vi "Initialize Queues and Buffers.vi"(4 "XNET Cluster":refnum<k21>, 5 "initial values":dbl[](array[numeric]), 6 "XNET Database":refnum<k21>, 7 "scaling information":T6, 8 "error in":errorcluster, 10 "stop notifier":refnum<notifier>, 11 "J1939 init data":T1={"CAN Port"="", "CAN Termination"=0, "timing"={"tb to j1939 queue timeout"=100, "j1939 to tb queue timeout"=100, "dtc loop period (ms)"=100, "CAN in loop period (ms)"=100, "process incoming queue timeout (ms)"=100, "Outgoing Write Decimation"=0, "process outgoing loop rate (ms)"=100, "periodic outgoing queue timeout (ms)"=10, "CAN out queue timeout (ms)"=100}, "database"={"BaudRate"=0, "CAN.IoMode"=0, "J1939 Network Address"=0, "Name"=0, "frames"=[]}} {"CAN Termination" items=["Off", "On"]}) -> (0 "error out":errorcluster, 3 "j1939 internals":T8={"J1939 XNET Settings"={"XNET Database"="", "XNET Cluster"="", "CAN port"="", "Baud rate [Bd]"=0, "J1939 Network Address"=0, "Name"=0, "Termination"=0}, "j1939 queues"={"Processed Outgoing"=refnum, "Process Outgoing"=refnum, "stop notifier"=refnum, "error queue"=refnum, "active dtc"=refnum, "processed inc"=refnum}, "fgv references"={"BAM Buffer"=refnum, "CM Buffer"=refnum, "CM Gen"=refnum, "BAM Gen"=refnum, "Address Claims"=refnum, "RQST"=refnum, "scaling lut"=refnum, "data lut"=refnum, "cyclic scheduler"=refnum}, "frame in"="", "frame out"="", "timing"={"tb to j1939 queue timeout"=100, "j1939 to tb queue timeout"=100, "dtc loop period (ms)"=100, "CAN in loop period (ms)"=100, "process incoming queue timeout (ms)"=100, "Outgoing Write Decimation"=0, "process outgoing loop rate (ms)"=0, "periodic outgoing queue timeout (ms)"=10, "CAN out queue timeout (ms)"=100}})   [LabVIEW 2013, in "J1939.lvlib"]
uses:
  J1939.lvlib
  API Types/Internal Data.ctl
  API Types/XNET Settings.ctl
  Users/Benjamin/Desktop/Tag bus J1939/J1939/RT Driver/J1939 Multi Packet Frame/_SubVIs/J1939 Setup Information Cluster.ctl
  API Types/CAN Outgoing Message Cluster.ctl
  Users/Benjamin/Desktop/Tag bus J1939/J1939/RT Driver/J1939 Multi Packet Frame/_SubVIs/J1939 Convert DTCs Cluster.ctl
  <vilib>/xnet/xnet.llb/XNET Frame CAN.ctl
  <vilib>/xnet/xnet.llb/XNET Frame Type CAN.ctl
  Users/Benjamin/Desktop/Tag bus J1939/J1939/RT Driver/J1939 Multi Packet Frame/_SubVIs/J1939 TP List References.ctl
  Users/Benjamin/Desktop/Tag bus J1939/J1939/RT Driver/J1939 Multi Packet Frame/_SubVIs/J1939 BAM Buffer Connections List_Ref.ctl
  Users/Benjamin/Desktop/Tag bus J1939/J1939/RT Driver/J1939 Multi Packet Frame/_SubVIs/J1939 Connection Mode Generation Connection Ref.ctl
  Users/Benjamin/Desktop/Tag bus J1939/J1939/RT Driver/J1939 Multi Packet Frame/_SubVIs/J1939 BAM Generation Connections List_Ref.ctl
  LUTs/J1939 Address Table Reference.ctl
  Users/Benjamin/Desktop/Tag bus J1939/J1939/RT Driver/J1939 Multi Packet Frame/_SubVIs/J1939 RQST Lookup Table Reference.ctl
  LUTs/J1939 Conversion Lookup Table Reference.ctl
  LUTs/J1939 Data Lookup Table Reference.ctl
  LUTs/Cyclic Frame Scheduler Lut Reference.ctl
  Configuration/TypeDefs/timing configuration.ctl
  API Types/Scaling Initialization.ctl
  Users/Benjamin/Desktop/Tag bus J1939/J1939/RT Driver/SubVIs/CD Conversion Lookup Table Parameters Cluster.ctl
  Configuration/TypeDefs/initialization data.ctl
  Configuration/TypeDefs/J1939 db.ctl
  Configuration/TypeDefs/J1939 db frame.ctl
  Configuration/TypeDefs/J1939 db signal.ctl
  <vilib>/xnet/xnet.llb/XNET Create Session (Frame Input Stream).vi
  <vilib>/xnet/xnet.llb/XNET Create Session (Frame Output Stream).vi
  <resource>/objmgr/xnet.rc
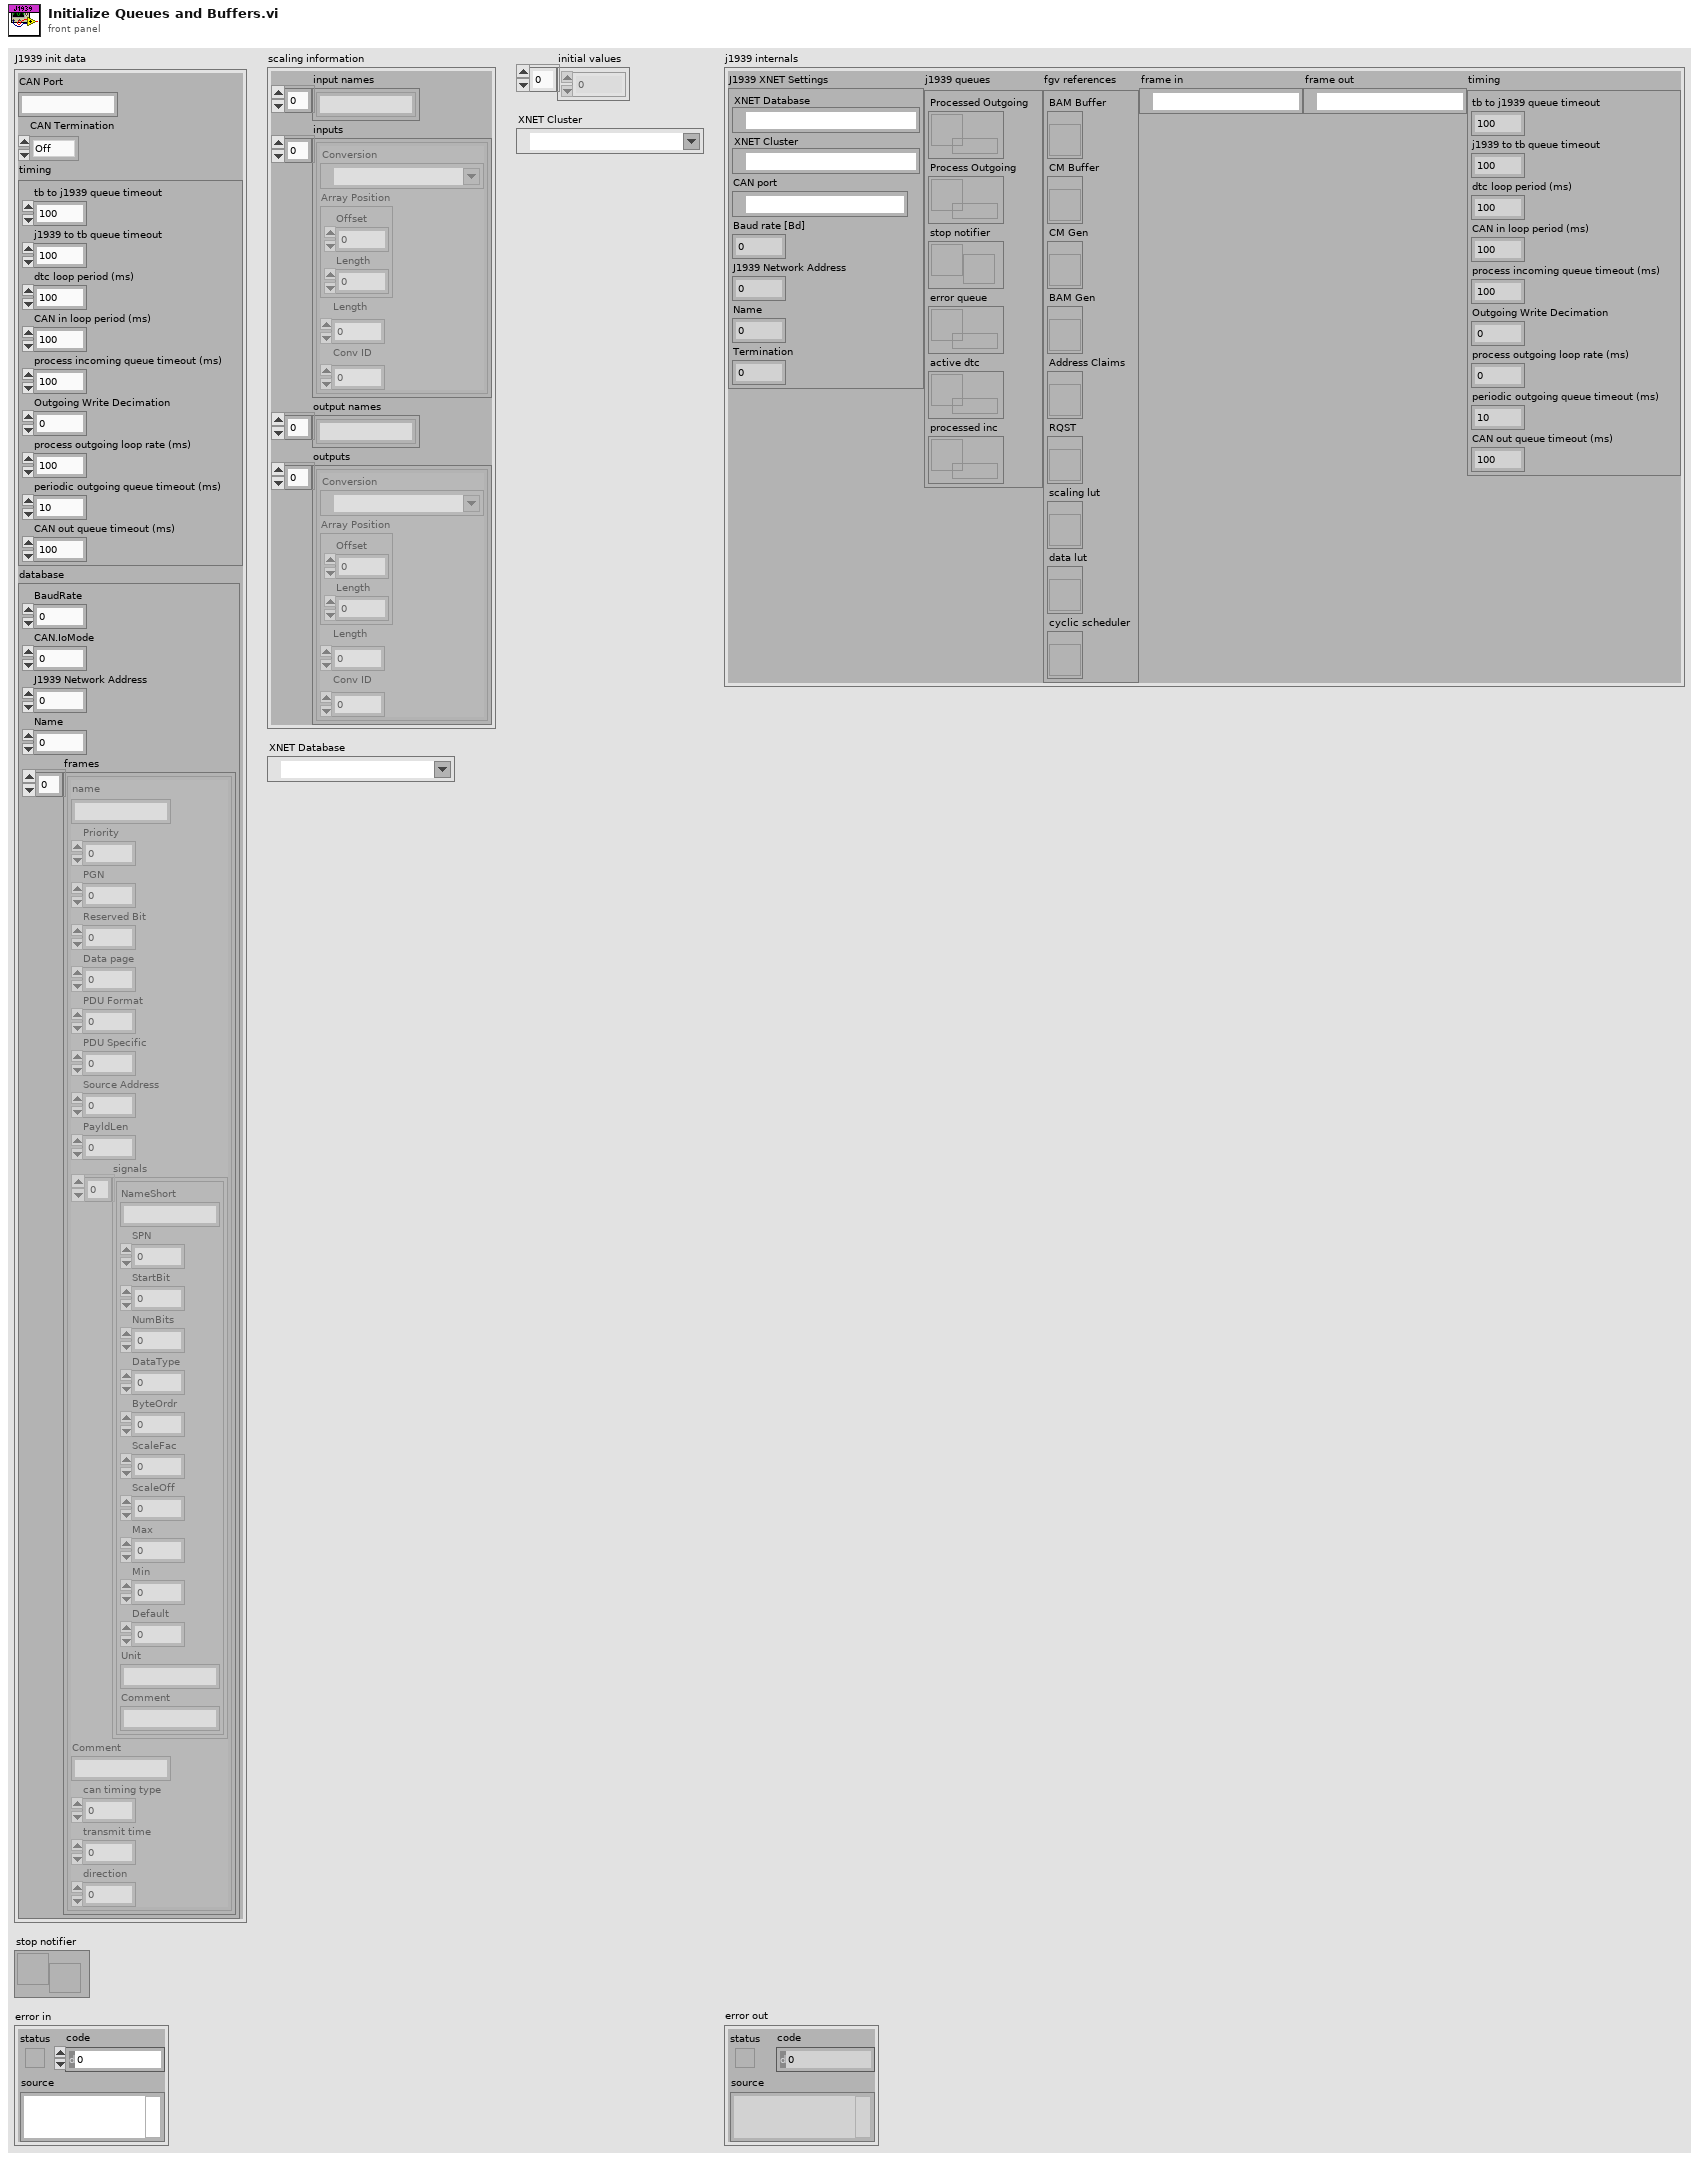
[diagram p1: front panel]
types:
  T1 = typedef "J1939.lvlib/initialization data.ctl" = cluster{"CAN Port":string, "CAN Termination":u32, "timing":T2, "database":T3}
  T2 = typedef "J1939.lvlib/timing configuration.ctl" = cluster{"tb to j1939 queue timeout":i32, "j1939 to tb queue timeout":i32, "dtc loop period (ms)":i32, "CAN in loop period (ms)":i32, "process incoming queue timeout (ms)":i32, "Outgoing Write Decimation":u32, "process outgoing loop rate (ms)":i32, "periodic outgoing queue timeout (ms)":i32, "CAN out queue timeout (ms)":i32}
  T3 = typedef "J1939.lvlib/J1939 db.ctl" = cluster{"BaudRate":u32, "CAN.IoMode":u32, "J1939 Network Address":u8, "Name":u64, "frames":T4[]}
  T4 = typedef "J1939.lvlib/J1939 db frame.ctl" = cluster{"name":string, "Priority":u8, "PGN":u32, "Reserved Bit":u8, "Data page":u8, "PDU Format":u8, "PDU Specific":u8, "Source Address":u8, "PayldLen":u32, "signals":T5[], "Comment":string, "can timing type":u32, "transmit time":dbl, "direction":u16}
  T5 = typedef "J1939.lvlib/J1939 db signal.ctl" = cluster{"NameShort":string, "SPN":i32, "StartBit":u32, "NumBits":u32, "DataType":u32, "ByteOrdr":u32, "ScaleFac":dbl, "ScaleOff":dbl, "Max":dbl, "Min":dbl, "Default":dbl, "Unit":string, "Comment":string}
  T6 = typedef "J1939.lvlib/scaling initialization.ctl" = cluster{"input names":string[], "inputs":T7[], "output names":string[], "outputs":T7[]}
  T7 = typedef "J1939.lvlib/CD Conversion Lookup Table Parameters Cluster.ctl" = cluster{"Conversion":refnum<k21>, "Array Position":cluster{"Offset":u32, "Length":u32}, "Length":u32, "Conv ID":u32}
  T8 = typedef "J1939.lvlib/Internal Data.ctl" = cluster{"J1939 XNET Settings":T9, "j1939 queues":T10, "fgv references":T11, "frame in":refnum<k21>, "frame out":refnum<k21>, "timing":T2}
  T9 = typedef "J1939.lvlib/XNET settings.ctl" = cluster{"XNET Database":refnum<k21>, "XNET Cluster":refnum<k21>, "CAN port":refnum<k21>, "Baud rate [Bd]":u32, "J1939 Network Address":u8, "Name":u64, "Termination":u32}
  T10 = typedef "J1939.lvlib/J1939 Setup Information Cluster.ctl" = cluster{"Processed Outgoing":refnum<queue>, "Process Outgoing":refnum<queue>, "stop notifier":refnum<notifier>, "error queue":refnum<queue>, "active dtc":refnum<queue>, "processed inc":refnum<queue>}
  T11 = typedef "J1939.lvlib/J1939 TP List References.ctl" = cluster{"BAM Buffer":T12, "CM Buffer":T12, "CM Gen":T13, "BAM Gen":T14, "Address Claims":T15, "RQST":T16, "scaling lut":T17, "data lut":T18, "cyclic scheduler":T19}
  T12 = typedef "J1939.lvlib/J1939 BAM Buffer Connections List_Ref.ctl" = refnum<vi>
  T13 = typedef "J1939.lvlib/J1939 Connection Mode Generation Connection Ref.ctl" = refnum<vi>
  T14 = typedef "J1939.lvlib/J1939 BAM Generation Connections List_Ref.ctl" = refnum<vi>
  T15 = typedef "J1939.lvlib/J1939 Address Table Reference.ctl" = refnum<vi>
  T16 = typedef "J1939.lvlib/J1939 RQST Lookup Table Reference.ctl" = refnum<vi>
  T17 = typedef "J1939.lvlib/J1939 Conversion Lookup Table Reference.ctl" = refnum<vi>
  T18 = typedef "J1939.lvlib/J1939 Data Lookup Table Reference.ctl" = refnum<vi>
  T19 = typedef "J1939.lvlib/cyclic frame scheduler lut reference.ctl" = refnum<vi>
  T20 = typedef "J1939.lvlib/J1939 Convert DTCs Cluster.ctl" = cluster{"Lamps":cluster{"Malfunction Indicator":u8, "Red Stop":u8, "Amber Warning":u8, "Protect Lamp":u8}, "DTCs":cluster{"SPN":u32, "FMI":u8, "Occurrance":u8}[], "Active?":bool, "Address":u8, "timestamp":timestamp}
  T21 = typedef "XNET Frame CAN.ctl" = cluster{"timestamp":timestamp, "payload":u8[], "identifier":u32, "type":T22, "extended?":bool, "echo?":bool}
  T22 = typedef "XNET Frame Type CAN.ctl" = u8
  T23 = typedef "J1939.lvlib/CAN Outgoing Message Cluster.ctl" = cluster{"Identifier":u32, "Data":u8[]}
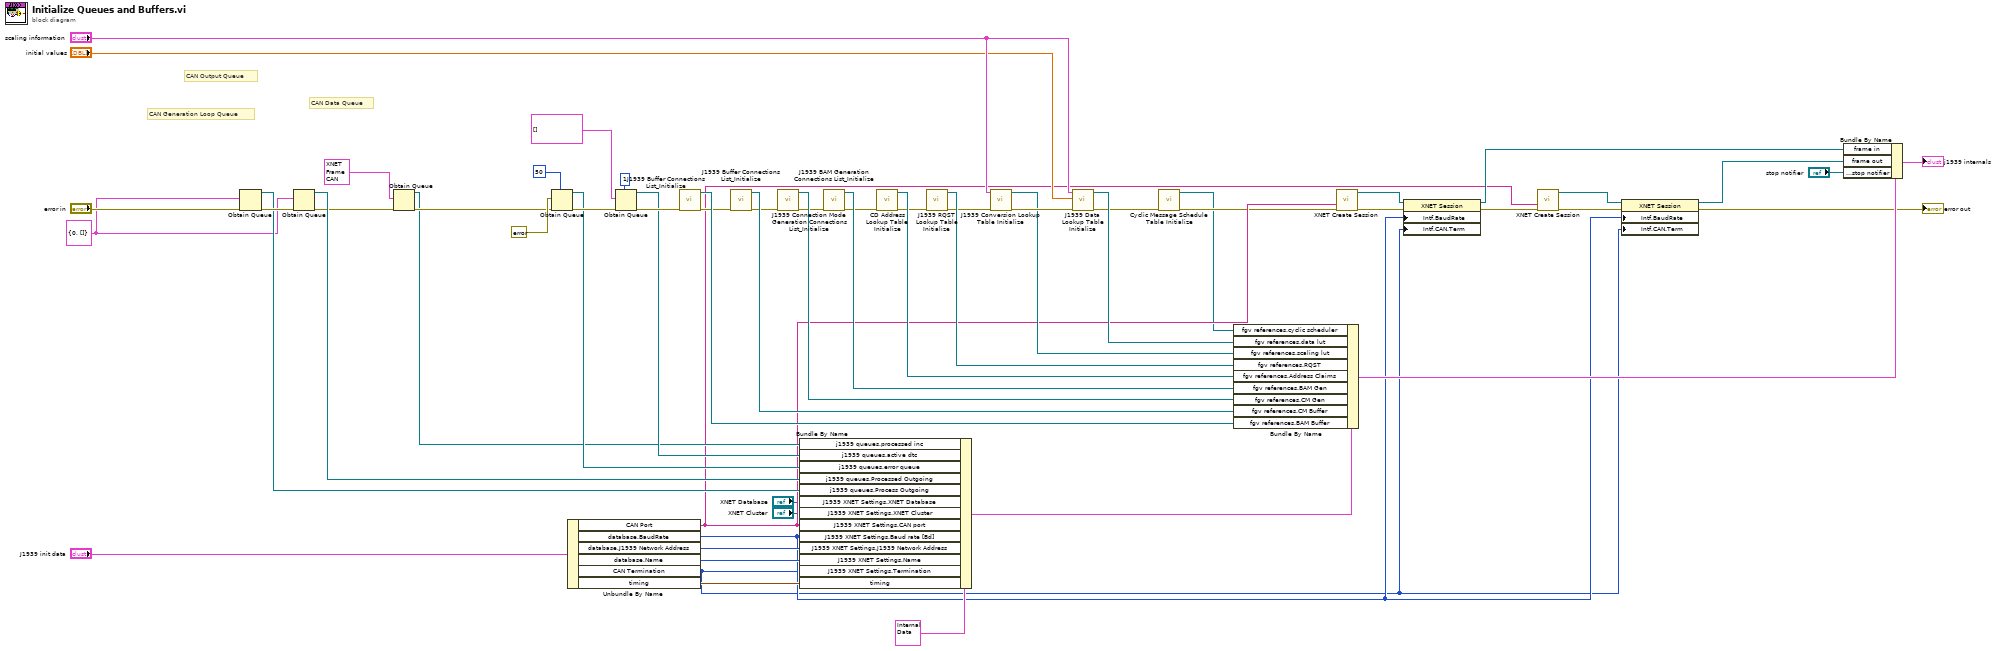
[diagram p0: block diagram]
diagram:
  w18 = T23 {"Identifier"=0, "Data"=[]} ("Data to Send")
  # "CAN Generation Loop Queue"
  # "CAN Output Queue"
  # "CAN Data Queue"
  n1 = Obtain Queue(element data type=w18, error in (no error)="error in") -> (queue out=w56:refnum<queue>, error out=w58:errorcluster)  [unwired: 3 in, 1 out]
  n2 = Obtain Queue(element data type=w18, error in (no error)=w58) -> (queue out=w57:refnum<queue>, error out=w17:errorcluster)  [unwired: 3 in, 1 out]
  n3 = Obtain Queue(element data type=T21 {"timestamp"=timestamp(0 s since 1904-01-01), "payload"=[], "identifier"=0, "type"=0, "extended?"=FALSE, "echo?"=FALSE} ("CAN frame"), error in (no error)=w17) -> (queue out=w14:refnum<queue>, error out=w16:errorcluster)  [unwired: 3 in, 1 out]
  n4 = Obtain Queue(max queue size (-1, unlimited)=50, element data type=errorcluster {"status"=FALSE, "code"=0, "source"=""} ("error out"), error in (no error)=w16) -> (queue out=w25:refnum<queue>, error out=w26:errorcluster)  [unwired: 2 in, 1 out]
  n5 = Unbundle By Name("J1939 init data") -> ("CAN Port"=w8:string, "database.BaudRate"=w7:u32, "database.J1939 Network Address"=w11:u8, "database.Name"=w10:u64, "CAN Termination"=w6:u32, "timing"=w9:T2)
  n6 = Obtain Queue(max queue size (-1, unlimited)=1, element data type=T20[] [] ("Responses"), error in (no error)=w26) -> (queue out=w19:refnum<queue>, error out=w22:errorcluster)  [unwired: 2 in, 1 out]
  n7 = call "J1939 Buffer Connections List_Initialize.vi"("error in (no error)"=w22) -> ("error out"=w54:errorcluster, "reference out"=w55:T12)  [unwired: 9 in]
  n8 = call "J1939 Buffer Connections List_Initialize.vi"("error in (no error)"=w54) -> ("error out"=w52:errorcluster, "reference out"=w53:T12)  [unwired: 9 in]
  n9 = call "J1939 Connection Mode Generation Connections List_Initialize.vi"("error in (no error)"=w52) -> ("error out"=w50:errorcluster, "CM Gen Ref out"=w51:T13)  [unwired: 9 in]
  n10 = Bundle By Name(cluster=T8 {"J1939 XNET Settings"={"XNET Database"="", "XNET Cluster"="", "CAN port"="", "Baud rate [Bd]"=0, "J1939 Network Address"=0, "Name"=0, "Termination"=0}, "j1939 queues"={"Processed Outgoing"=refnum, "Process Outgoing"=refnum, "stop notifier"=refnum, "error queue"=refnum, "active dtc"=refnum, "processed inc"=refnum}, "fgv references"={"BAM Buffer"=refnum, "CM Buffer"=refnum, "CM Gen"=refnum, "BAM Gen"=refnum, "Address Claims"=refnum, "RQST"=refnum, "scaling lut"=refnum, "data lut"=refnum, "cyclic scheduler"=refnum}, "frame in"="", "frame out"="", "timing"={"tb to j1939 queue timeout"=0, "j1939 to tb queue timeout"=0, "dtc loop period (ms)"=0, "CAN in loop period (ms)"=0, "process incoming queue timeout (ms)"=0, "Outgoing Write Decimation"=0, "process outgoing loop rate (ms)"=0, "periodic outgoing queue timeout (ms)"=0, "CAN out queue timeout (ms)"=0}} ("internal data"), "j1939 queues.processed inc"=w14, "j1939 queues.active dtc"=w19, "j1939 queues.error queue"=w25, "j1939 queues.Processed Outgoing"=w57, "j1939 queues.Process Outgoing"=w56, "J1939 XNET Settings.XNET Database"="XNET Database", "J1939 XNET Settings.XNET Cluster"="XNET Cluster", "J1939 XNET Settings.CAN port"=w8, "J1939 XNET Settings.Baud rate [Bd]"=w7, "J1939 XNET Settings.J1939 Network Address"=w11, "J1939 XNET Settings.Name"=w10, "J1939 XNET Settings.Termination"=w6, "timing"=w9) -> (w43:T8)
  n11 = call "J1939 BAM Generation Connections List_Initialize.vi"("error in (no error)"=w50) -> ("error out"=w48:errorcluster, "BAM Gen"=w49:T14)  [unwired: 9 in]
  n12 = call "CD Address Lookup Table Initialize.vi"("error in (no error)"=w48) -> ("error out"=w46:errorcluster, "ref"=w47:T15)  [unwired: 9 in]
  n13 = call "J1939 RQST Lookup Table Initialize.vi"("error in (no error)"=w46) -> ("error out"=w32:errorcluster, "reference out"=w45:T16)  [unwired: 9 in]
  n14 = call "J1939 Conversion Lookup Table Initialize.vi"("error in"=w32, "scaling information"="scaling information") -> ("error out"=w33:errorcluster, "vi reference"=w30:T17)  [unwired: 8 in]
  n15 = call "J1939 Data Lookup Table Initialize.vi"("error in (no error)"=w33, "initial values"="initial values", "channel information"="scaling information") -> ("error out"=w5:errorcluster, "vi reference"=w31:T18)  [unwired: 7 in]
  n16 = call "Cyclic Message Schedule Table Initialize.vi"("error in"=w5) -> ("error out"=w4:errorcluster, "reference out"=w3:T19)  [unwired: 9 in]
  n17 = Bundle By Name(cluster=w43, "fgv references.cyclic scheduler"=w3, "fgv references.data lut"=w31, "fgv references.scaling lut"=w30, "fgv references.RQST"=w45, "fgv references.Address Claims"=w47, "fgv references.BAM Gen"=w49, "fgv references.CM Gen"=w51, "fgv references.CM Buffer"=w53, "fgv references.BAM Buffer"=w55) -> (w37:T8)
  n18 = call-poly <vilib>:"XNET Create Session.vi"("interface"=w8, "error in (no error)"=w4) -> ("session out"=w42:refnum<k21>, "error out"=w41:errorcluster)  [unwired: 12 out]
  n19 = property class="XNET Session"(reference=w42, error in=w41, "Intf.BaudRate"=w7, "Intf.CAN.Term"=w6) -> (reference out=w36:refnum<k21>, error out=w38:errorcluster)
  n20 = call-poly <vilib>:"XNET Create Session.vi"("interface"=w8, "error in (no error)"=w38) -> ("session out"=w40:refnum<k21>, "error out"=w39:errorcluster)  [unwired: 12 out]
  n21 = property class="XNET Session"(reference=w40, error in=w39, "Intf.BaudRate"=w7, "Intf.CAN.Term"=w6) -> (reference out=w35:refnum<k21>, error out=→"error out":errorcluster)
  n22 = Bundle By Name(cluster=w37, "frame in"=w36, "frame out"=w35, "j1939 queues.stop notifier"="stop notifier") -> (→"j1939 internals":T8)
